vi "SendSetDataSendParameters.vi"(8 "error in (no error)":errorcluster, 10 "send parameters":T1, 11 "Qbus in":refnum<class "Qbus.lvclass">) -> (0 "error out":errorcluster, 3 "Qbus out":refnum<class "Qbus.lvclass">)   [LabVIEW 2017, in "ServerComm.lvlib"]
uses:
  <vilib>/addons/InsightCM/Devices/Shared/Common/ServerComm/ServerComm.lvlib
  <vilib>/addons/Qbus/Qbus.lvclass
  <vilib>/addons/InsightCM/Devices/Shared/Common/ServerComm/controls/DataSendParameters.ctl
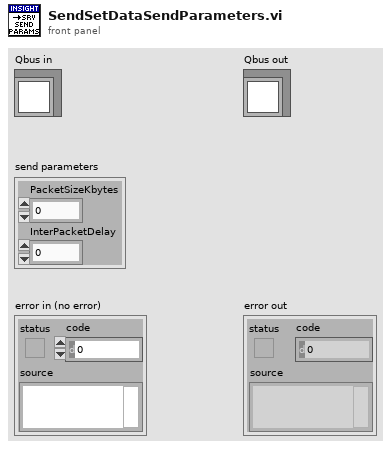
[diagram p1: front panel]
types:
  T1 = typedef "ServerComm.lvlib/DataSendParameters.ctl" = cluster{"PacketSizeKbytes":i32, "InterPacketDelay":i32}
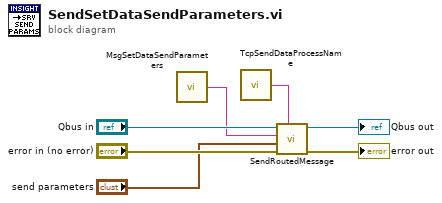
[diagram p0: block diagram]
diagram:
  n1 = call <vilib>:"MsgSetDataSendParameters.vi"() -> ("message name"=w1:string)  [unwired: 5 in]
  n2 = call <vilib>:"TcpSendDataProcessName.vi"() -> ("process name"=w3:string)  [unwired: 5 in]
  n3 = call <vilib>:"SendRoutedMessage.vi"("listener process"=w3, "error in (no error)"="error in (no error)", "message value"="send parameters", "message name"=w1, "Qbus in"="Qbus in") -> ("error in (no error)"=→"error out":errorcluster, "Qbus out"=→"Qbus out":refnum<class "Qbus.lvclass">)  [unwired: 5 in]
